vi "Timer_Elasped.vi"(8 "error in (no error)":errorcluster, 10 "ElapsedTime to test (ms)":u32, 11 "Timer in":refnum<class "Timer.lvclass">) -> (0 "error out":errorcluster, 1 "Elapsed ?":bool, 2 "ElapsedTime (ms)":u32, 3 "Timer out":refnum<class "Timer.lvclass">)   [LabVIEW 2020, in "Timer.lvclass"]
doc: "Measure Elapsed time and test if time is finished"
uses:
  Timer.lvclass
  Timer.lvclass/Timer.ctl
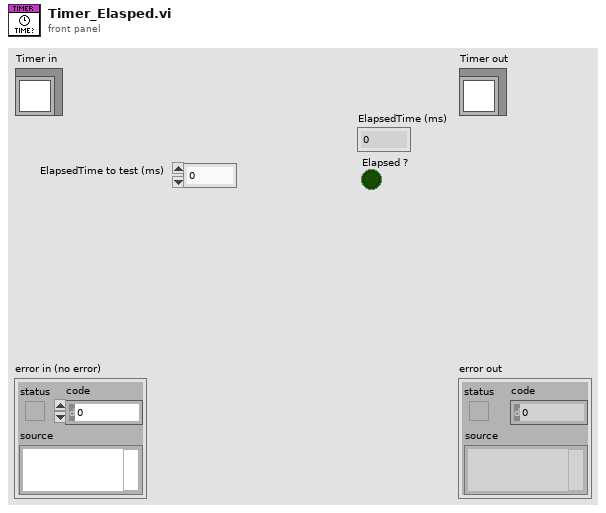
[diagram p1: front panel]
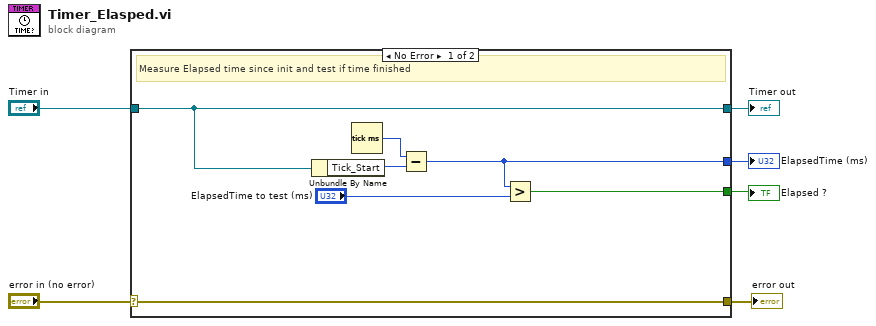
[diagram p0: block diagram]
diagram:
  n1 = case shown="No Error" "error in (no error)" {
    selector: "error in (no error)" -> [w13 w15]
    tunnel: [w13 w15] -> w5
    tunnel: [w12 w14] -> w3
    tunnel: "Timer in" -> [w12 w14]
    tunnel: [w9 _] -> w2
    tunnel: [w7 _] -> w1
    frame No Error {
      # "Measure Elapsed time since init and test if time finished"
      n2 = Unbundle By Name(w12) -> ("Tick_Start"=w11:u32)
      n3 = Tick Count (ms)() -> (millisecond timer value=w10:u32)
      n4 = Subtract(x=w10, y=w11) -> (x-y=w9:u32)
      n5 = Greater?(x=w9, y="ElapsedTime to test (ms)") -> (0:w7:bool)
    }
    frame Error {
    }
  }
  "error out" <- w5
  "Timer out" <- w3
  "ElapsedTime (ms)" <- w2
  "Elapsed ?" <- w1
